vi "Aurora Config No Framework.vi"(0 "address space.lvclass:address space instruction in":T2, 5 "input valid (instruction)":bool) -> (4 "response out":T1, 6 "done":bool, 8 "ready for input":bool)   [LabVIEW 2019]
doc: "Manages the mapping between AXI4-Lite and the Instruction Framework and performs the bus transactions.\n\n<B>Input Parameters</B>\n\n<B>niInstr AXI4-Lite - FXP32 address - fxp32 data v1 FPGA in</B> is a reference to the class used to communicate.\n\n<B>abort</B> aborts the current data transaction. Currently unsupported.\n\n<B>address space.lvclass:address space instruction in</B> specifies the instruction to be written.\n\n<B>address space.lvclass:address space instruction in.address</B> specifies the address of the instruction to be written.\n\n<B>address space.lvclass:address space instruction in.data</B> specifies the instruction data to be written.\n\n<B>address space.lvclass:address space instruction in.read</B> is true for Read instructions and false for Write instructions.\n\n<B>input valid (instruction)</B> is true if the instruction on the current clock cycle is valid.\n\n<B>Output Parameters</B>\n\n<B>response out</B> is the response from the bus. This parameter is valid only if 'done' returns true.\n\n<B>response out.data</B> is the data of the response.\n\n<B>response out.error</B> is true if there was an error as part of the response.\n\n<B>done</B> indicates whether the received 'response out' is valid.\n\n<B>ready for input</B> indicates whether the bus is ready to accept more data."
uses:
  <vilib>/eio/EIONode/EIONode.xnode
  <vilib>/rvi/eio/common/nirviEmuTemplateMethod_errors.vi
  <instrlib>/_niInstr/Instruction Framework/v1/FPGA/Typedefs/Response.ctl
  <instrlib>/_niInstr/Instruction Framework/v1/FPGA/Typedefs/niInstr Instruction Framework v1 FPGA.lvlib
  <instrlib>/_niInstr/Instruction Framework/v1/FPGA/Interfaces/Address Space/Address Space Instruction.ctl
  <instrlib>/_niInstr/Instruction Framework/v1/FPGA/Interfaces/Address Space/Address Space.lvclass
  <instrlib>/_niInstr/Basic Elements/v1/FPGA/niInstr Basic Elements v1 FPGA.lvlib
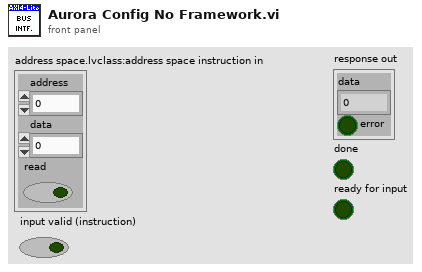
[diagram p1: front panel]
types:
  T1 = typedef "niInstr Instruction Framework v1 FPGA.lvlib/Response.ctl" = cluster{"data":u64, "error":bool}
  T2 = typedef "niInstr Instruction Framework Interfaces v1 FPGA.lvlib/Address Space.lvclass/Address Space Instruction.ctl" = cluster{"address":u32, "data":u64, "read":bool}
  T3 = enum16{"Send Write Address and Write Data", "Receive Write Response"}
  T4 = enum16{"Initialize", "Wait for Instruction", "Read", "Write"}
  T5 = typedef "AXI4-Lite Address Space.lvclass/AXI4-Lite State Machine State.ctl" = enum16{"Initialize", "Wait for Instruction", "Read", "Write"}
  T6 = typedef "AXI4-Lite Address Space.lvclass/AXI4-Lite Read State.ctl" = enum16{"Send Read Address", "Receive Read Data"}
  T7 = typedef "AXI4-Lite Address Space.lvclass/AXI4-Lite Write State.ctl" = enum16{"Send Write Address and Write Data", "Receive Write Response"}
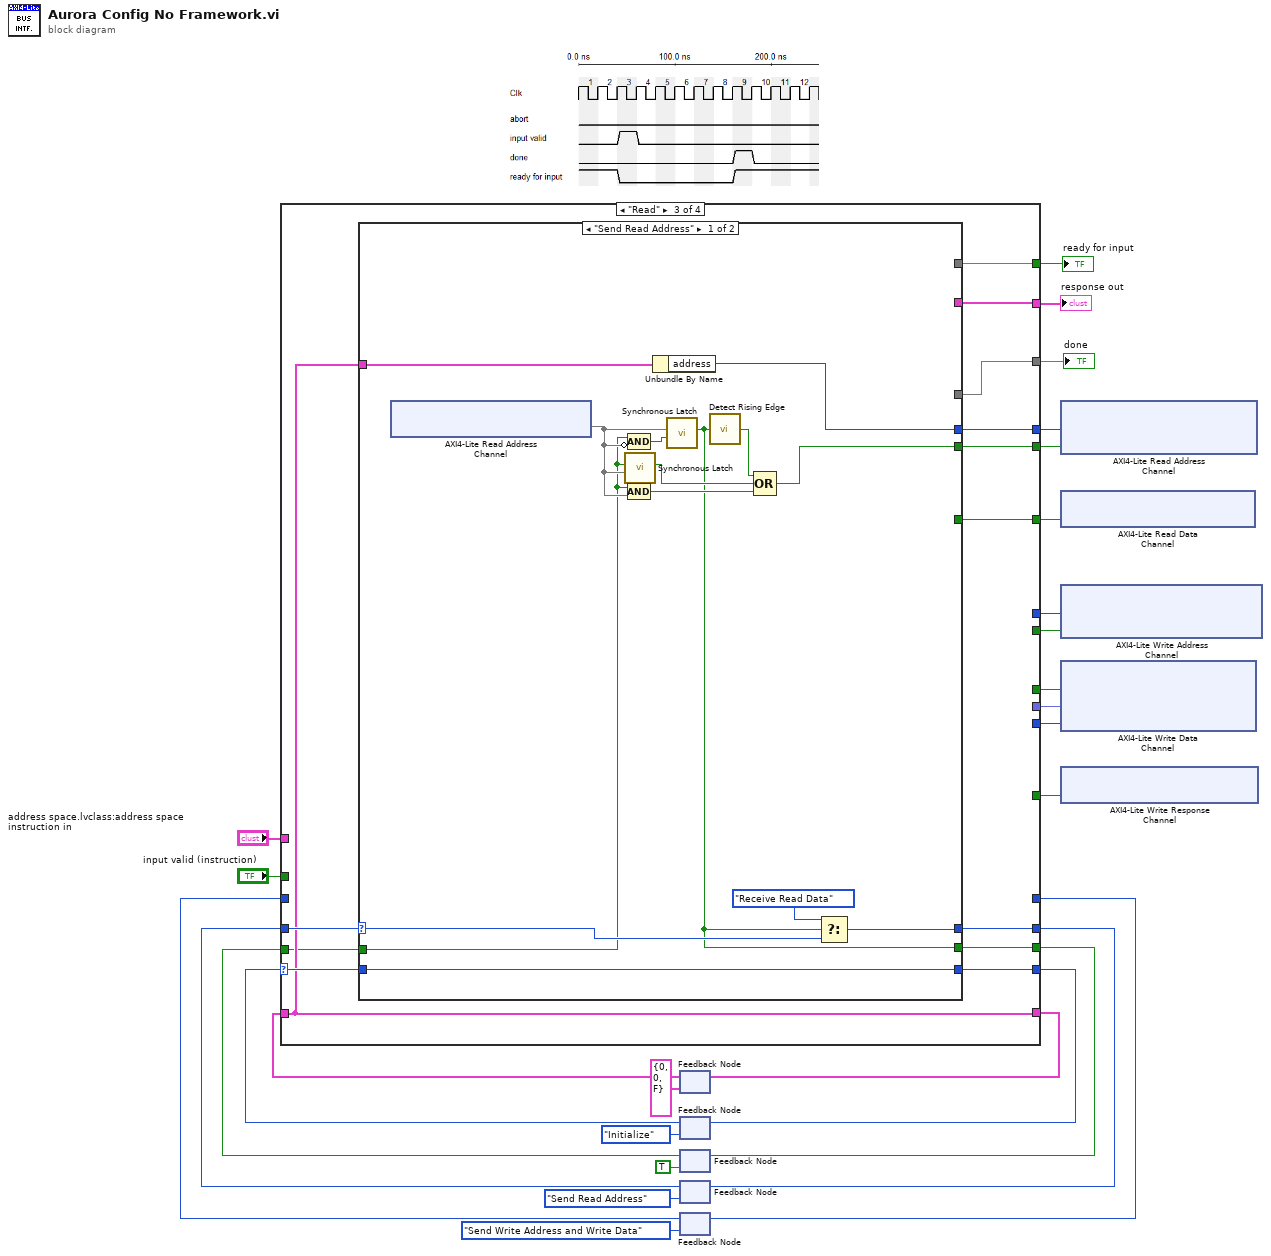
[diagram p0: block diagram]
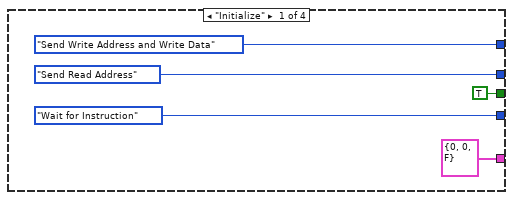
[diagram p2: hidden frame]
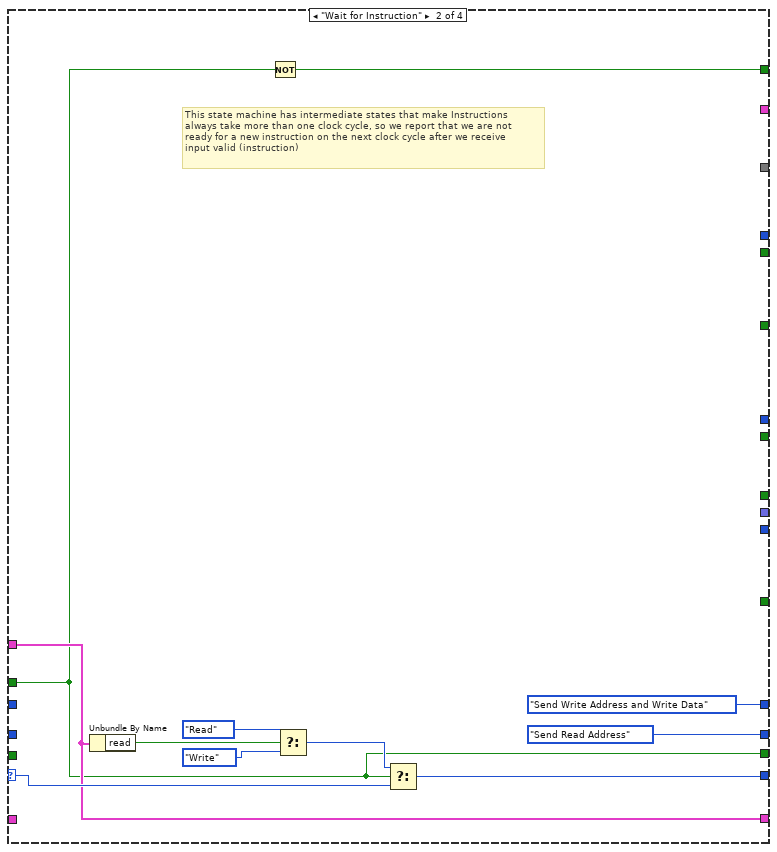
[diagram p3: hidden frame]
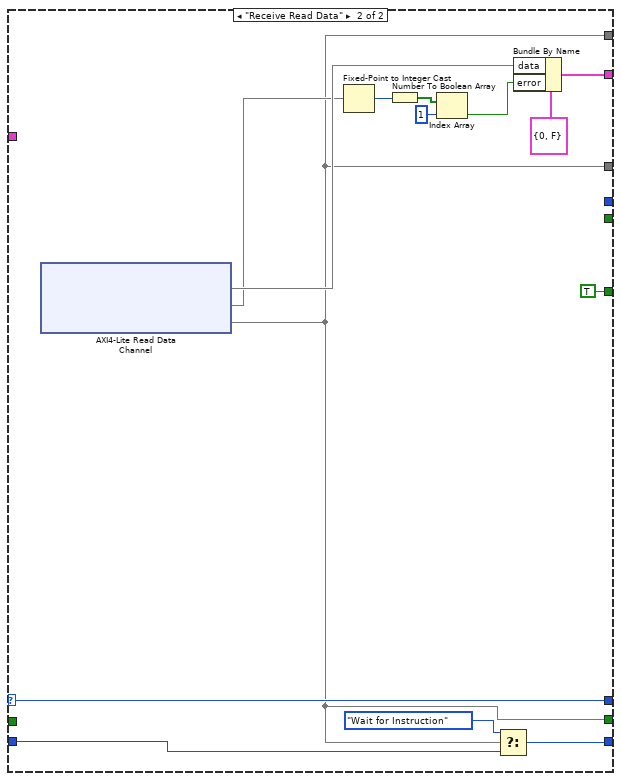
[diagram p4: hidden frame]
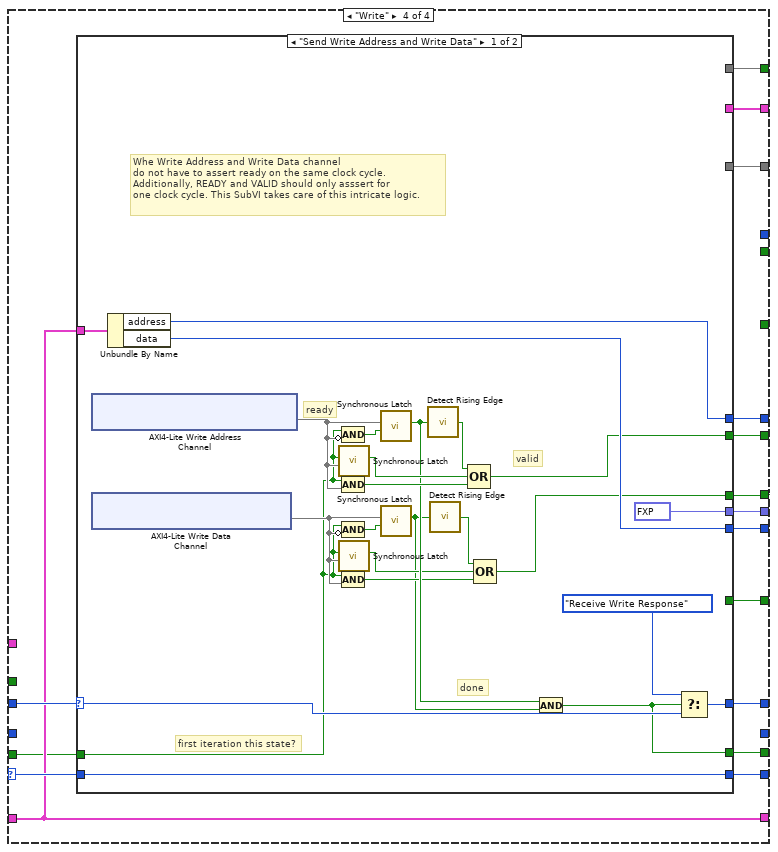
[diagram p5: hidden frame]
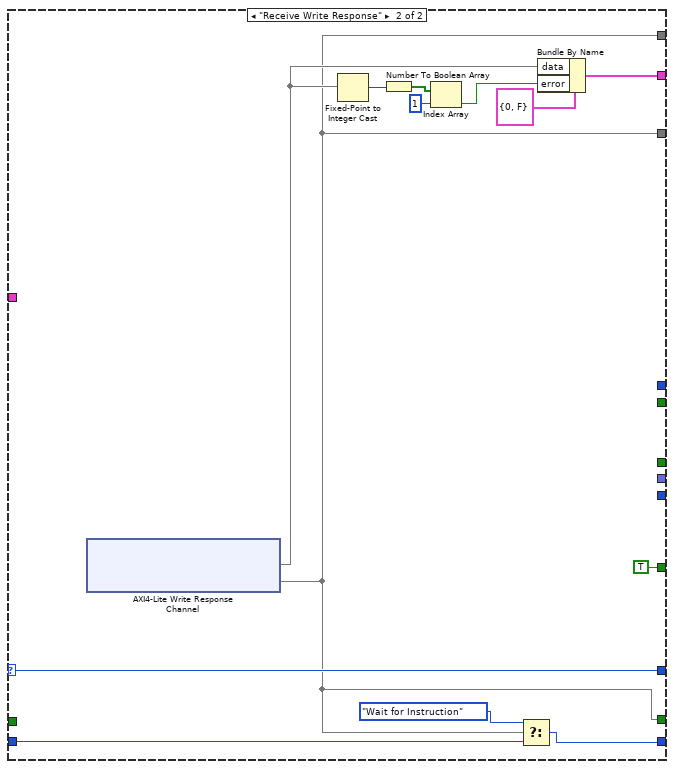
[diagram p6: hidden frame]
diagram:
  n1 = feedback #1(T2 {"address"=0, "data"=0, "read"=FALSE} ("instruction")) -> (w24:T2)
  n2 = feedback #2(T4."Initialize") -> (w4:T5)
  n3 = feedback #3(TRUE) -> (w2:bool)
  n4 = feedback #4(enum16{"Send Read Address", "Receive Read Data"}."Send Read Address") -> (w26:T6)
  n5 = feedback #5(T3."Send Write Address and Write Data" ("Enum")) -> (w25:T7)
  n6 = case shown="\"Read\"" w4 {
    selector: w4 -> [_ w42 w55 w98]
    tunnel: "address space.lvclass:address space instruction in" -> [_ w38 _ _]
    tunnel: "input valid (instruction)" -> [_ w35 _ _]
    tunnel: [T2 {"address"=0, "data"=0, "read"=FALSE} ("instruction") w38 w50 w90] -> w27
    tunnel: w24 -> [_ _ w50 w90]
    tunnel: [T4."Wait for Instruction" w41 w56 w97] -> w5
    tunnel: [enum16{"Send Read Address", "Receive Read Data"}."Send Read Address" enum16{"Send Read Address", "Receive Read Data"}."Send Read Address" w57 _] -> w7
    tunnel: w26 -> [_ _ w58 _]
    tunnel: [_ _ w54 w99] -> w10
    tunnel: [_ _ w53 w100] -> w28
    tunnel: [T3."Send Write Address and Write Data" ("Enum") T3."Send Write Address and Write Data" ("Enum") _ w101] -> w6
    tunnel: w25 -> [_ _ _ w102]
    tunnel: [_ _ _ w96] -> w19
    tunnel: [_ _ _ w95] -> w14
    tunnel: [_ _ w52 _] -> w18
    tunnel: [_ _ w51 _] -> w17
    tunnel: [_ _ _ w94] -> w16
    tunnel: [_ _ w49 _] -> w15
    tunnel: [_ _ _ w93] -> w13
    tunnel: [_ _ _ w92] -> w12
    tunnel: [_ _ _ w91] -> w11
    tunnel: [_ w36 w48 w89] -> w9
    tunnel: w2 -> [_ _ w46 w88]
    tunnel: [TRUE ("I/O Item") w35 w47 w87] -> w3
    frame "Initialize" {
    }
    frame "Wait for Instruction" {
      # "This state machine has intermediate states that make Instructions \nalways take more than one clock cycle, so we report that we are not \nready for a new instruction on the next clock cycle after we receive\ninput valid (instruction)"
      n7 = Unbundle By Name(w38) -> ("read"=w45:bool)
      n8 = Not(x=w35) -> (.not. x?=w36:bool)
      n9 = Select(t=T4."Read", s=w45, f=T4."Write") -> (s? t:f=w44:T4)
      n10 = Select(t=w44, s=w35, f=w42) -> (s? t:f=w41:T5)
    }
    frame "Read" {
      n11 = case shown="\"Send Read Address\"" w58 {
        selector: w58 -> [w72 w86]
        tunnel: w50 -> [w67 _]
        tunnel: [w69 w86] -> w57
        tunnel: [w60 _] -> w52
        tunnel: [w70 w85] -> w56
        tunnel: w55 -> [w70 w84]
        tunnel: [_ w74] -> w54
        tunnel: [_ w82] -> w53
        tunnel: [_ TRUE ("I/O Item")] -> w51
        tunnel: [w68 _] -> w49
        tunnel: [_ w74] -> w48
        tunnel: [w59 w74] -> w47
        tunnel: w46 -> [w61 _]
        frame "Send Read Address" {
          n12 = xnode "AXI4-Lite Read Address Channel"() -> ("7902R IO Socket\\s_axi_arready"=w62)  [unwired: 1 in, 1 out]
          n13 = call <instrlib>:"Synchronous Latch.vi"("clear"=w62, "set"=w61) -> ("out"=w66:bool)  [unwired: 9 in]
          n14 = Compound Arithmetic op=AND(w61, invert w62) -> (w65:bool)
          n15 = Compound Arithmetic op=AND(w61, w62) -> (w64:bool)
          n16 = Unbundle By Name(w67) -> ("address"=w68:u32)
          n17 = call <instrlib>:"Synchronous Latch.vi"("clear"=w65, "set"=w62) -> ("out"=w59:bool)  [unwired: 9 in]
          n18 = call <instrlib>:"Detect Rising Edge.vi"("signal"=w59) -> ("edge detected"=w63:bool)  [unwired: 14 in]
          n19 = Compound Arithmetic op=OR(w63, w66, w64) -> (w60:bool)
          n20 = Select(t=enum16{"Send Read Address", "Receive Read Data"}."Receive Read Data", s=w59, f=w72) -> (s? t:f=w69:T6)
        }
        frame "Receive Read Data" {
          n21 = xnode "AXI4-Lite Read Data Channel"() -> ("7902R IO Socket\\s_axi_rdata"=w81, "7902R IO Socket\\s_axi_rresp"=w77, "7902R IO Socket\\s_axi_rvalid"=w74)  [unwired: 3 in, 3 out]
          n22 = Fixed-Point to Integer Cast(1:w77) -> (0:w79:u8)
          n23 = Number To Boolean Array(number=w79) -> (Boolean array=w78:bool[])
          n24 = Index Array(array=w78, index=1) -> (element=w76:bool)
          n25 = Select(t=T4."Wait for Instruction", s=w74, f=w84) -> (s? t:f=w85:T5)
          n26 = Bundle By Name(cluster=T1 {"data"=0, "error"=FALSE} ("response"), "data"=w81, "error"=w76) -> (w82:T1)
        }
      }
    }
    frame "Write" {
      n27 = case shown="\"Send Write Address and Write Data\"" w102 {
        selector: w102 -> [w126 w134]
        tunnel: [w112 _] -> w96
        tunnel: [w106 _] -> w95
        tunnel: [w125 w134] -> w101
        tunnel: w90 -> [w123 _]
        tunnel: [_ w138] -> w100
        tunnel: [_ w128] -> w99
        tunnel: w98 -> [w122 w137]
        tunnel: [w122 w136] -> w97
        tunnel: [_ TRUE ("I/O Item")] -> w94
        tunnel: [fxp<+,4,4> 15.0 ("blk_mem_gen_v7_3 1\\s_axi_wstrb") _] -> w93
        tunnel: [w120 _] -> w92
        tunnel: [w119 _] -> w91
        tunnel: [_ w128] -> w89
        tunnel: w88 -> [w104 _]
        tunnel: [w118 w128] -> w87
        frame "Send Write Address and Write Data" {
          # "ready"
          # "first iteration this state?"
          # "done"
          # "valid"
          # "Whe Write Address and Write Data channel\ndo not have to assert ready on the same clock cycle.\nAdditionally, READY and VALID should only asssert for \none clock cycle. This SubVI takes care of this intricate logic."
          n28 = xnode "AXI4-Lite Write Address Channel"() -> ("7902R IO Socket\\s_axi_awready"=w113)  [unwired: 1 in, 1 out]
          n29 = xnode "AXI4-Lite Write Data Channel"() -> ("7902R IO Socket\\s_axi_wready"=w105)  [unwired: 1 in, 1 out]
          n30 = Unbundle By Name(w123) -> ("address"=w120:u32, "data"=w119:u64)
          n31 = call <instrlib>:"Synchronous Latch.vi"("clear"=w113, "set"=w104) -> ("out"=w117:bool)  [unwired: 9 in]
          n32 = call <instrlib>:"Synchronous Latch.vi"("clear"=w105, "set"=w104) -> ("out"=w110:bool)  [unwired: 9 in]
          n33 = Compound Arithmetic op=AND(w104, invert w113) -> (w116:bool)
          n34 = Compound Arithmetic op=AND(w104, w113) -> (w115:bool)
          n35 = Compound Arithmetic op=AND(w104, invert w105) -> (w109:bool)
          n36 = Compound Arithmetic op=AND(w104, w105) -> (w108:bool)
          n37 = call <instrlib>:"Synchronous Latch.vi"("clear"=w116, "set"=w113) -> ("out"=w111:bool)  [unwired: 9 in]
          n38 = call <instrlib>:"Synchronous Latch.vi"("clear"=w109, "set"=w105) -> ("out"=w103:bool)  [unwired: 9 in]
          n39 = call <instrlib>:"Detect Rising Edge.vi"("signal"=w111) -> ("edge detected"=w114:bool)  [unwired: 14 in]
          n40 = call <instrlib>:"Detect Rising Edge.vi"("signal"=w103) -> ("edge detected"=w107:bool)  [unwired: 14 in]
          n41 = Compound Arithmetic op=OR(w114, w117, w115) -> (w112:bool)
          n42 = Compound Arithmetic op=OR(w107, w110, w108) -> (w106:bool)
          n43 = And(x=w111, y=w103) -> (x .and. y?=w118:bool)
          n44 = Select(t=T3."Receive Write Response", s=w118, f=w126) -> (s? t:f=w125:T7)
        }
        frame "Receive Write Response" {
          n45 = xnode "AXI4-Lite Write Response Channel"() -> ("7902R IO Socket\\s_axi_bresp"=w130, "7902R IO Socket\\s_axi_bvalid"=w128)  [unwired: 2 in, 2 out]
          n46 = Fixed-Point to Integer Cast(1:w130) -> (0:w133:u8)
          n47 = Number To Boolean Array(number=w133) -> (Boolean array=w132:bool[])
          n48 = Index Array(array=w132, index=1) -> (element=w129:bool)
          n49 = Select(t=T4."Wait for Instruction", s=w128, f=w137) -> (s? t:f=w136:T5)
          n50 = Bundle By Name(cluster=T1 {"data"=0, "error"=FALSE} ("response"), "data"=w130, "error"=w129) -> (w138:T1)
        }
      }
    }
  }
  "response out" <- w28
  "done" <- w10
  "ready for input" <- w9
  n51 = feedback-in #1(w27) -> ()
  n52 = feedback-in #2(w5) -> ()
  n53 = feedback-in #3(w3) -> ()
  n54 = feedback-in #4(w7) -> ()
  n55 = feedback-in #5(w6) -> ()
  n56 = xnode "AXI4-Lite Read Address Channel"("7902R IO Socket\\s_axi_araddr"=w15, "7902R IO Socket\\s_axi_arvalid"=w18) -> ()  [unwired: 2 in, 2 out]
  n57 = xnode "AXI4-Lite Read Data Channel"("7902R IO Socket\\s_axi_rready"=w17) -> ()  [unwired: 1 in, 1 out]
  n58 = xnode "AXI4-Lite Write Address Channel"("7902R IO Socket\\s_axi_awaddr"=w12, "7902R IO Socket\\s_axi_awvalid"=w19) -> ()  [unwired: 2 in, 2 out]
  n59 = xnode "AXI4-Lite Write Data Channel"("7902R IO Socket\\s_axi_wvalid"=w14, "7902R IO Socket\\s_axi_wstrb"=w13, "7902R IO Socket\\s_axi_wdata"=w11) -> ()  [unwired: 3 in, 3 out]
  n60 = xnode "AXI4-Lite Write Response Channel"("7902R IO Socket\\s_axi_bready"=w16) -> ()  [unwired: 1 in, 1 out]
